vi "Main On Compile Action VI.vi"(8 "error in (no error)":errorcluster, 11 "Device Item Ref in":T1 format="%.0x") -> (0 "error out":errorcluster)   [LabVIEW 2017, in "Ballard 1553 System Explorer.lvlib"]
uses:
  Ballard 1553 System Explorer.lvlib
  <vilib>/NI Veristand/Custom Device API/Custom Device Item Ref.ctl
  Shared/Controls and Global/Compiled.Settings.ctl
  Shared/Controls and Global/RT Channel.ctl
  Shared/Controls and Global/RT BC.ctl
  Shared/Controls and Global/RT Message.ctl
  Shared/Controls and Global/RT messageType.ctl
  Shared/Controls and Global/RT CWD1.ctl
  Shared/Controls and Global/RT CWD2.ctl
  <vilib>/NI Veristand/Custom Device API/Data Reference.ctl
  <vilib>/NI Veristand/Custom Device API/Block Data Reference.ctl
  Shared/Controls and Global/RT Remote Terminal.ctl
  Shared/Controls and Global/RT Remote Terminal_rtMode.ctl
  Shared/Controls and Global/RT Remote Terminal_RT subAddress.ctl
  Shared/Controls and Global/RT Remote Terminal_RT direction.ctl
  Shared/Controls and Global/RT Remote Terminal_RT Mode Code.ctl
  <vilib>/NI Veristand/Custom Device API/Set Item Property (Variant).vi
  <vilib>/NI VeriStand/Custom Device API/Custom Device API.lvlib
  <vilib>/NI/NIVS Inline Async API/_Data Access System Explorer/Data Access System Explorer.lvlib
  Shared/Ballard 1553 Shared.lvlib
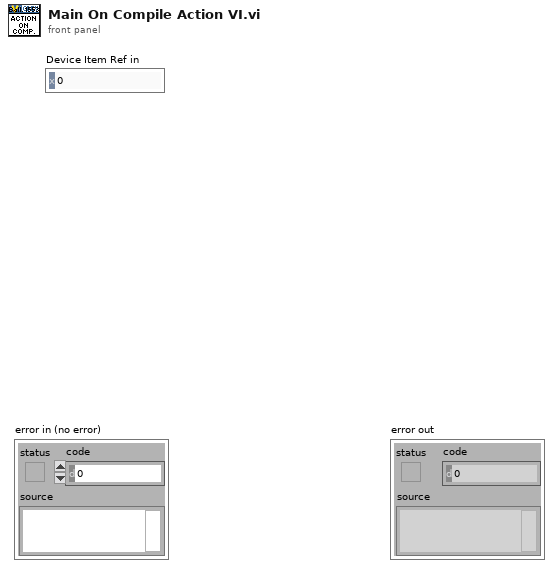
[diagram p1: front panel]
types:
  T1 = typedef "Custom Device API.lvlib/Custom Device Item Ref.ctl" = u64
  T2 = typedef "Ballard 1553 Shared.lvlib/Compiled.Settings.ctl" = cluster{"Name":string, "channels":T3[]}
  T3 = typedef "Ballard 1553 Shared.lvlib/RT Channel.ctl" = cluster{"name":string, "hardWare Channel Number":u16, "BC":T4, "RTs":T11[]}
  T4 = typedef "Ballard 1553 Shared.lvlib/RT BC.ctl" = cluster{"ID":i32, "name":string, "Command Channels Refs":T1[], "messages":T5[], "Acyclic Frames Trigger Channels Refs":T1[], "Acyclic Frames Names":string[]}
  T5 = typedef "Ballard 1553 Shared.lvlib/RT Message.ctl" = cluster{"Name":string, "messageType":T6, "CWD1":T7, "CWD2":T8, "Status Channel Data Refs":T9[], "Words Item Refs":T1[], "Words Block Data Refs":T10[], "Words Values Array":u16[], "Timestamp Channel Data Reference":T9, "ID":i32, "Timestamp?":bool, "Data Words?":bool, "Status Channel Ref?":bool}
  T6 = typedef "Ballard 1553 Shared.lvlib/RT messageType.ctl" = enum16{"BC to RT", "RT to BC", "RT to RT", "MC (Rx)", "MC (Tx)"}
  T7 = typedef "Ballard 1553 Shared.lvlib/RT CWD1.ctl" = cluster{"TA (RT)":i8, "SA":i8, "Mode Code":i8, "Words Count":i8}
  T8 = typedef "Ballard 1553 Shared.lvlib/RT CWD2.ctl" = cluster{"TA (RT)":i8, "SA":i8, "Words (WC)":i8}
  T9 = typedef "Custom Device API.lvlib/Data Reference.ctl" = i32
  T10 = typedef "Custom Device API.lvlib/Block Data Reference.ctl" = cluster{"Data Reference":T9, "Offset":u64, "Length":u64}
  T11 = typedef "Ballard 1553 Shared.lvlib/RT Remote Terminal.ctl" = cluster{"ID":i32, "name":string, "RT Address":i32, "rtMode":T12, "Command Channels Refs":T1[], "Status Channel Data Reference":T9, "subAddresses":T13[], "Mode Codes":T15[]}
  T12 = typedef "Ballard 1553 Shared.lvlib/RT Remote Terminal_rtMode.ctl" = enum16{"Simulate", "Monitor", "Disable"}
  T13 = typedef "Ballard 1553 Shared.lvlib/RT Remote Terminal_RT subAddress.ctl" = cluster{"name":string, "subAddress":i8, "direction":T14, "Timestamp Channel Data Reference":T9, "Words Values Array":u16[], "Words Block Data Refs":T10[], "Words Item Refs":T1[], "ID":i32, "Timestamp?":bool, "Data Words?":bool}
  T14 = typedef "Ballard 1553 Shared.lvlib/RT Remote Terminal_RT direction.ctl" = enum16{"Tx", "Rx"}
  T15 = typedef "Ballard 1553 Shared.lvlib/RT Remote Terminal_RT Mode Code.ctl" = cluster{"name":string, "direction":T14, "Timestamp Channel Data Reference":T9, "Words Values Array":u16[], "Words Block Data Refs":T10[], "Words Item Refs":T1[], "ID":i32, "Timestamp?":bool, "Data Words?":bool, "Code Number":i32}
  T16 = typedef "Custom Device API.lvlib/Custom Device Item Info.ctl" = cluster{"Name":string, "Is Channel":bool, "GUID":string, "Is Waveform":bool}
  T17 = cluster{"Name":string, "Type":enum16{"Output/Write", "Input/Read", "Input/ReadWrite"}, "VS Refs":T1[]}
  T18 = cluster{"Name":string, "Type":enum16{"Output/Write", "Input/Read", "Input/ReadWrite"}, "VS Refs":T1[]}[]
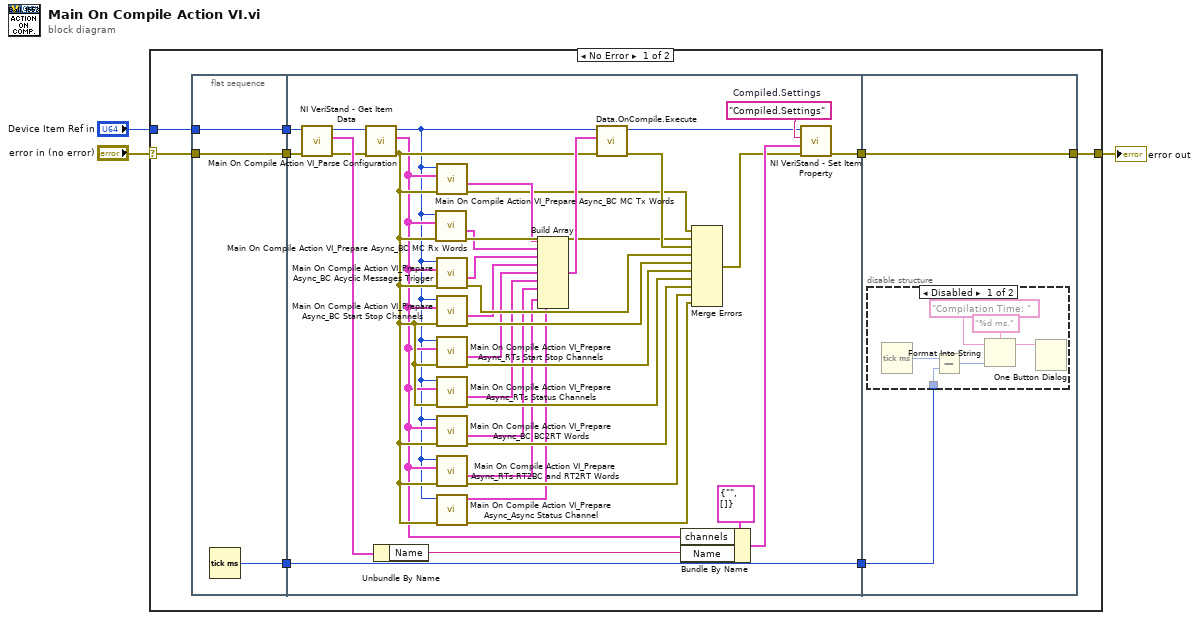
[diagram p0: block diagram]
diagram:
  n1 = case shown="No Error" "error in (no error)" {
    selector: "error in (no error)" -> [w11 w59]
    tunnel: [w9 w59] -> w3
    tunnel: "Device Item Ref in" -> [w10 _]
    frame No Error {
      n2 = flat-sequence {
        tunnel: w11 -> [w13]
        tunnel: w10 -> [w14]
        tunnel: [w14] -> w8
        tunnel: [w13] -> w7
        tunnel: [w12] -> w6
        tunnel: w8 -> [w47]
        tunnel: w7 -> [w48]
        tunnel: w6 -> [w50]
        tunnel: [w50] -> w5
        tunnel: [w44] -> w4
        tunnel: [w52] -> w9
        tunnel: w5 -> [w51]
        tunnel: w4 -> [w52]
        frame #0 {
          n3 = Tick Count (ms)() -> (millisecond timer value=w12:u32)
        }
        frame #1 {
          w42 = "Compiled.Settings"  # Compiled.Settings
          n4 = call <vilib>:"NI VeriStand - Get Item Data.vi"("error in (no error)"=w48, "Item Ref in"=w47) -> ("error out"=w39:errorcluster, "Item Info"=w49:T16, "Item Ref out"=w38:T1)  [unwired: 6 in, 1 out]
          n5 = call "Main On Compile Action VI_Parse Configuration.vi"("error in (no error)"=w39, "Item Ref in"=w38) -> ("error out"=w18:errorcluster, "Channels"=w17:T3[], "Section Ref out"=w16:T1)  [unwired: 7 in]
          n6 = Unbundle By Name(w49) -> ("Name"=w45:string)
          n7 = call "Main On Compile Action VI_Prepare Async_BC MC Rx Words.vi"("error in (no error)"=w18, "channels"=w17, "Item Ref In"=w16) -> ("error out"=w28:errorcluster, "Group"=w20:T17)  [unwired: 5 in, 2 out]
          n8 = call "Main On Compile Action VI_Prepare Async_BC MC Tx Words.vi"("error in (no error)"=w18, "channels"=w17, "Item Ref In"=w16) -> ("error out"=w15:errorcluster, "Group"=w19:T17)  [unwired: 5 in, 2 out]
          n9 = call "Main On Compile Action VI_Prepare Async_BC Acyclic Messages Trigger.vi"("error in (no error)"=w18, "channels"=w17, "Item Ref In"=w16) -> ("error out"=w29:errorcluster, "Group"=w21:T17)  [unwired: 5 in, 2 out]
          n10 = call "Main On Compile Action VI_Prepare Async_BC Start Stop Channels.vi"("error in (no error)"=w18, "channels"=w17, "Item Ref In"=w16) -> ("error out"=w37:errorcluster, "Group"=w27:T17)  [unwired: 5 in, 2 out]
          n11 = call "Main On Compile Action VI_Prepare Async_RTs Start Stop Channels.vi"("error in (no error)"=w18, "channels"=w17, "Item Ref In"=w16) -> ("error out"=w35:errorcluster, "Group"=w26:T17)  [unwired: 5 in, 2 out]
          n12 = call "Main On Compile Action VI_Prepare Async_RTs Status Channels.vi"("error in (no error)"=w18, "channels"=w17, "Item Ref In"=w16) -> ("error out"=w34:errorcluster, "Group"=w25:T17)  [unwired: 5 in, 2 out]
          n13 = call "Main On Compile Action VI_Prepare Async_BC BC2RT Words.vi"("error in (no error)"=w18, "channels"=w17, "Item Ref In"=w16) -> ("error out"=w33:errorcluster, "Group"=w24:T17)  [unwired: 5 in, 2 out]
          n14 = call "Main On Compile Action VI_Prepare Async_RTs RT2BC and RT2RT Words.vi"("error in (no error)"=w18, "channels"=w17, "Item Ref In"=w16) -> ("error out"=w32:errorcluster, "Group"=w23:T17)  [unwired: 5 in, 2 out]
          n15 = call "Main On Compile Action VI_Prepare Async_Async Status Channel.vi"("error in (no error)"=w18, "Item Ref"=w16) -> ("error out"=w31:errorcluster, "Async Status Channels Refs"=w22:T17)  [unwired: 8 in]
          n16 = Build Array(w19, w20, w21, w27, w26, w25, w24, w23, w22) -> (w36:T18)
          n17 = call <vilib>:"Data.OnCompile.Execute.vi"("error in"=w18, "VS Ref Groups"=w36, "Custom Device Ref"=w16) -> ("error out"=w30:errorcluster, "Custom Device Ref"=w40:T1)  [unwired: 7 in]
          n18 = Bundle By Name(cluster=T2 {"Name"="", "channels"=[]} ("Compiled.Settings"), "channels"=w17, "Name"=w45) -> (w46:T2)
          n19 = Merge Errors(w15, w28, w30, w29, w37, w35, w34, w33, w32, w31) -> (w41:errorcluster)
          n20 = call-poly <vilib>:"NI VeriStand - Set Item Property.vi"("error in (no error)"=w41, "Value"=w46, "Property Name"=w42, "Item Ref in"=w40) -> ("error out"=w44:errorcluster)  [unwired: 5 in, 2 out]
        }
        frame #2 {
          n21 = disable-structure shown="Disabled" {
            disable-tunnel: w51 -> [w57 _]
            frame Disabled {
              n22 = Tick Count (ms)() -> (millisecond timer value=w58:u32)
              n23 = Subtract(x=w58, y=w57) -> (x-y=w56:u32)
              n24 = Format Into String(format string="%d ms.", initial string="Compilation Time: ", w56) -> (resulting string=w55:string)  [unwired: 1 in, 1 out]
              n25 = One Button Dialog(message=w55) -> ()  [unwired: 1 in, 1 out]
            }
            frame Enabled {
            }
          }
        }
      }
    }
    frame Error {
    }
  }
  "error out" <- w3
